vi "Installer Post-Install Action.vi"   [LabVIEW 2020]
types:
  T1 = enum32{"Invalid", "Standard", "Closed", "Hidden", "Minimized", "Maximized"}
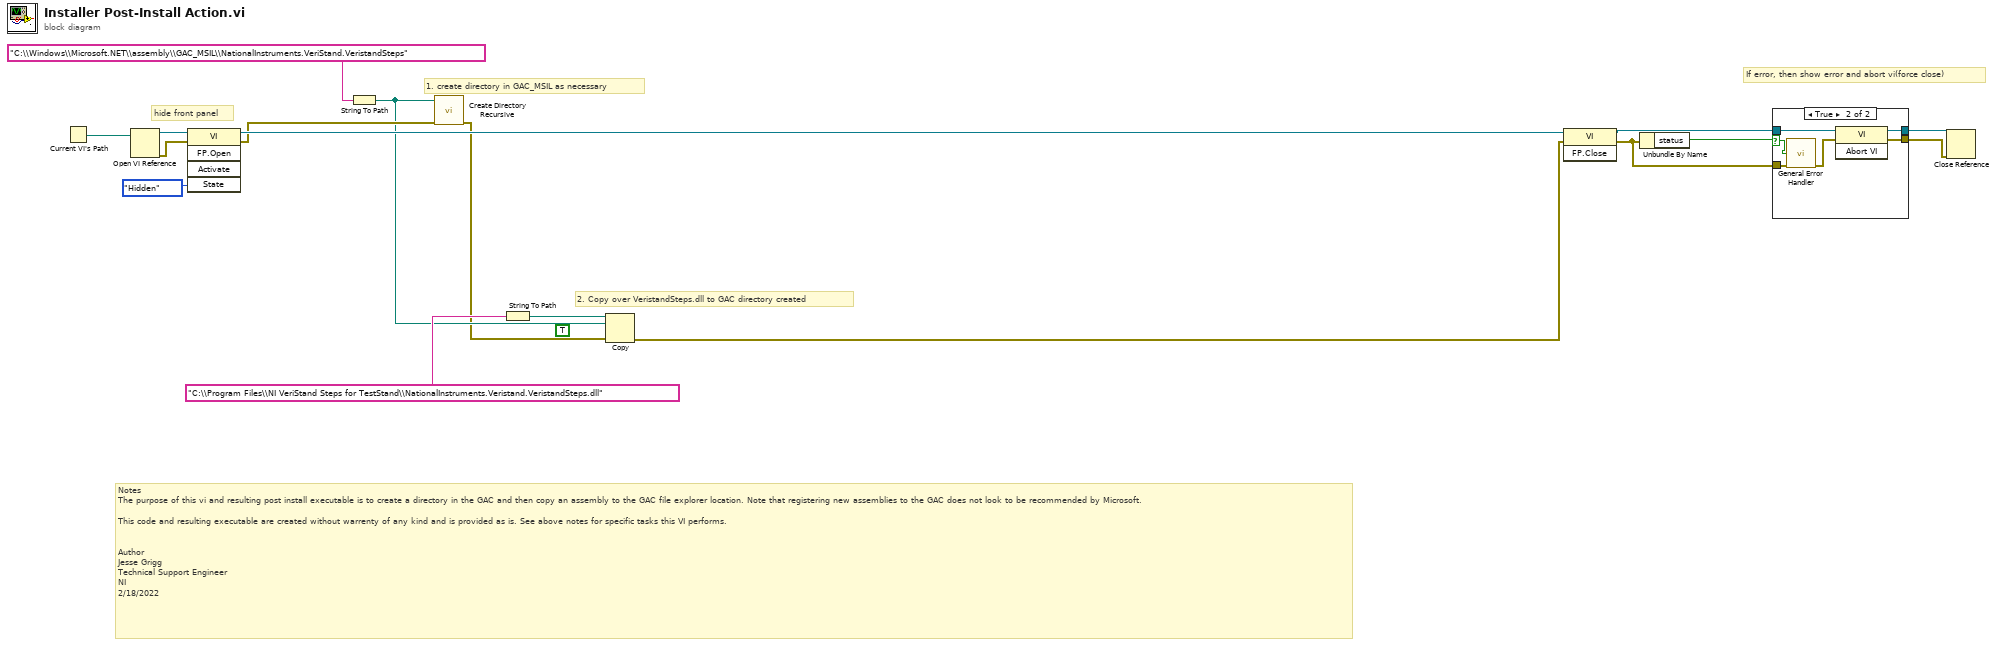
[diagram p0: block diagram]
diagram:
  (unwired) TRUE ("overwrite (F)")
  # "Notes\nThe purpose of this vi and resulting post install executable is to create a directory in the GAC and then copy an assembly to the GAC file explorer location. Note that registering new assemblies to the GAC does not look to be recommended by Microsoft.\n\nThis code and resulting executable are created without warrenty of any kind and is provided as is. See above notes for specific tasks this VI performs.\n\n\nAuthor\nJesse Grigg\nTechnical Support Engineer\nNI\n2/18/2022"
  # "2. Copy over VeristandSteps.dll to GAC directory created"
  # "1. create directory in GAC_MSIL as necessary"
  # "hide front panel"
  # "If error, then show error and abort vi(force close)"
  n1 = Current VI's Path() -> (path=w16:path)
  n2 = Open VI Reference(vi path=w16) -> (vi reference=w14:refnum<vi>, error out=w15:errorcluster)  [unwired: 5 in]
  n3 = invoke class="VI" method="FP.Open"(reference=w14, error in=w15, "State"=T1."Hidden") -> (reference out=w12:refnum<vi>, error out=w11:errorcluster)  [unwired: 2 in, 3 out]
  n4 = String To Path(string="C:\\Windows\\Microsoft.NET\\assembly\\GAC_MSIL\\NationalInstruments.VeriStand.VeristandSteps") -> (path=w3:path)
  n5 = call <vilib>:"Create Directory Recursive.vi"("error in (no error)"=w11, "directory"=w3) -> ("error out"=w2:errorcluster)  [unwired: 3 in, 2 out]
  n6 = String To Path(string="C:\\Program Files\\NI VeriStand Steps for TestStand\\NationalInstruments.Veristand.VeristandSteps.dll") -> (path=w4:path)
  n7 = Copy(8:w2, 10:w3, 11:w4) -> (0:w1:errorcluster)  [unwired: 2 in, 2 out]
  n8 = invoke class="VI" method="FP.Close"(reference=w12, error in=w1) -> (reference out=w8:refnum<vi>, error out=w6:errorcluster)  [unwired: 1 in, 1 out]
  n9 = Unbundle By Name(w6) -> ("status"=w9:bool)
  n10 = case shown="True" w9 {
    selector: w9 -> [_ w23]
    tunnel: w8 -> [w19 w25]
    tunnel: [w19 w24] -> w7
    tunnel: w6 -> [w18 w22]
    tunnel: [w18 w20] -> w5
    frame False {
    }
    frame True {
      n11 = call <vilib>:"General Error Handler.vi"("search ni.com link visible?(T)"=w23, "error in (no error)"=w22) -> ("error out"=w21:errorcluster)  [unwired: 9 in, 4 out]
      n12 = invoke class="VI" method="Abort VI"(reference=w25, error in=w21) -> (reference out=w24:refnum<vi>, error out=w20:errorcluster)  [unwired: 1 in, 1 out]
    }
  }
  n13 = Close Reference(reference=w7, error in (no error)=w5) -> ()  [unwired: 1 out]
